vi "Write ServerRequest.vi"(10 "ServerRequest":refnum<queue>, 11 "TCPConnectionHandler in":refnum<class "ConnectionHandler.lvclass">) -> (3 "TCPConnectionHandler out":refnum<class "ConnectionHandler.lvclass">)   [LabVIEW 2013, in "MQTT_Connection.lvlib" / "ConnectionHandler.lvclass"]
uses:
  ConnectionHandler.lvclass
  MQTT_Base/Base Class/Request -- cluster.ctl
  <vilib>/LabVIEW Open Source Project/MQTT Control Packets/Control Packets/ControlPacket/ControlPacket.lvclass
  MQTT_Base/Base Class/Response -- cluster.ctl
  ConnectionHandler.lvclass/ConnectionHandler.ctl
  MQTT_Base/Base Class/MQTT_Base.lvclass
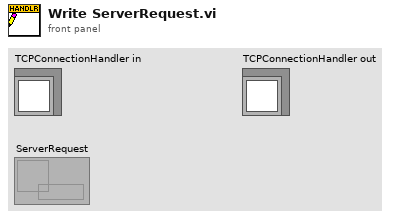
[diagram p1: front panel]
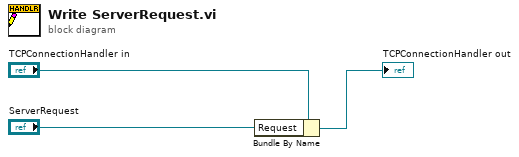
[diagram p0: block diagram]
diagram:
  n1 = Bundle By Name(cluster="TCPConnectionHandler in", "Request"="ServerRequest") -> (→"TCPConnectionHandler out":refnum<class "ConnectionHandler.lvclass">)
